vi "simx Set Object Orientation.vi"(6 "operationMode":i32, 7 "eulerAngles":sgl, 8 "error in (no error)":errorcluster, 9 "relativeToObjectHandle":i32, 10 "objectHandle":i32, 11 "clientID":i32) -> (0 "error out":errorcluster, 3 "function return":i32)   [LabVIEW 2019, in "PXL_V-REP.lvlib"]
doc: "EXTAPI_DLLEXPORT simxInt simxSetObjectOrientation(simxInt clientID,simxInt objectHandle,simxInt relativeToObjectHandle,const simxFloat* eulerAngles,simxInt operationMode);"
uses:
  PXL_V-REP.lvlib
  <userlib>/V-REP/remoteApi.dll
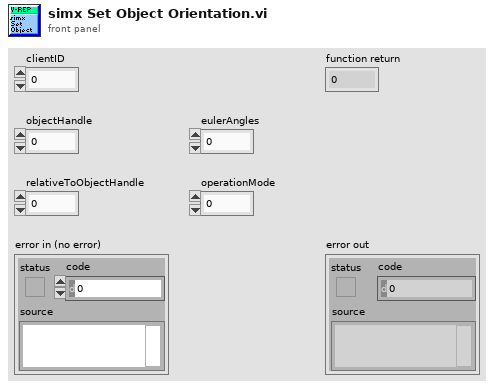
[diagram p1: front panel]
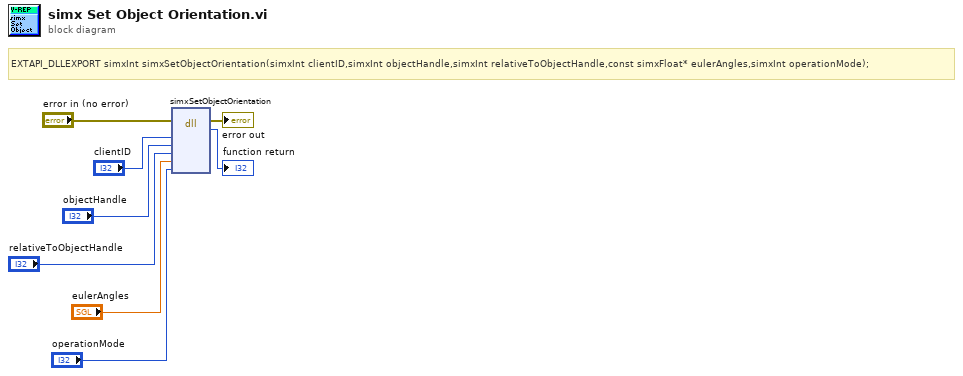
[diagram p0: block diagram]
diagram:
  # "EXTAPI_DLLEXPORT simxInt simxSetObjectOrientation(simxInt clientID,simxInt objectHandle,simxInt relativeToObjectHandle,const simxFloat* eulerAngles,simxInt operationMode);"
  n1 = dll-call lib="C:/Program Files (x86)/National Instruments/LabVIEW 2019/user.lib/V-REP/remoteApi.*" fn="simxSetObjectOrientation"(error in="error in (no error)", "clientID"="clientID", "objectHandle"="objectHandle", "relativeToObjectHandle"="relativeToObjectHandle", "eulerAngles"="eulerAngles", "operationMode"="operationMode") -> (error out=→"error out":errorcluster, →"function return":i32)  [unwired: 7 in, 1 out]
